vi "AO_mini_stage and shutter control.vi"() -> ()   [LabVIEW 2018]
panel:
  in  "2p shutter":refnum<k7>(container)
  in  "488 shutter":refnum<k7>(container)
  out "Numeric status":dbl
  in  "Flip Mirror":sgl(ring) items=["EMCCD Camera"=-5, "Wavefront sensor"=1]
  in  "stop":bool
  in  "baud rate (9600)":u32=9600
  in  "VISA resource name":refnum<visa-resource-name>="COM5"
  in  "Z step (10=1um)":dbl=2.0
  in  "up":bool
  in  "down":bool
  in  "XY step (10=1um)":u16=50
  in  "back":bool
  in  "front":bool
  in  "left":bool
  in  "right":bool
  # "Sample Stage"
  # "WF switch"
  # "Defocus: +"
  # "Tilt 1/X: +"
  # "Tilt 2/Y: +"
  # "EMCCD: -5"
  # "Wavefront Sensor: 1"
  # "WFS no tilt: X502, Y520 @EMCCD"
  # "Laser Shutter"
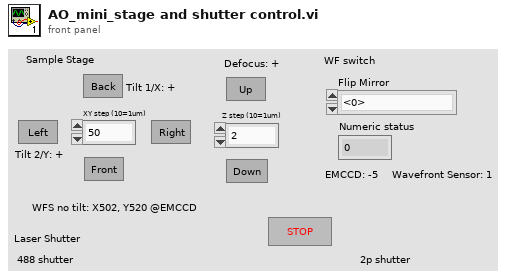
[diagram p1: front panel]
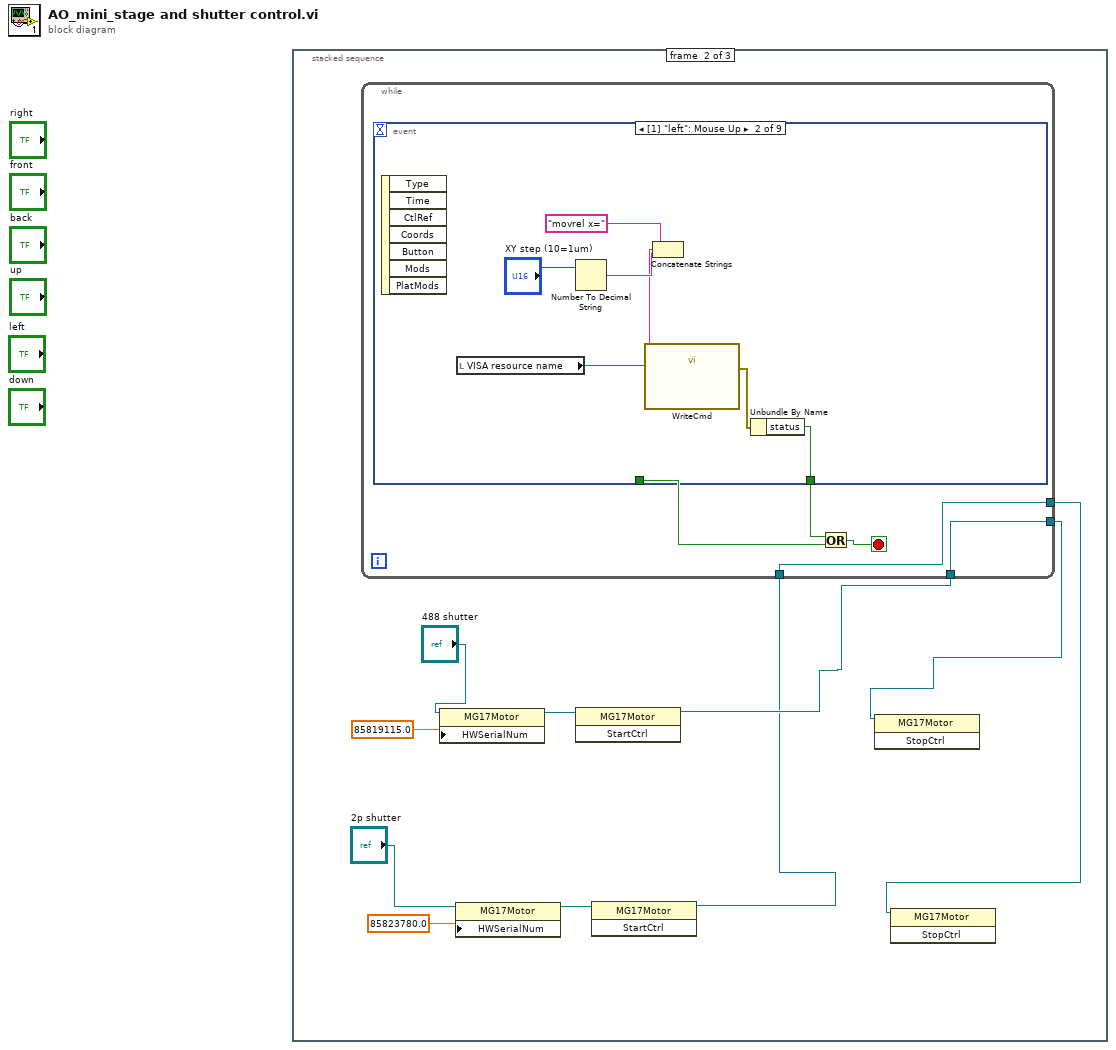
[diagram p0: block diagram]
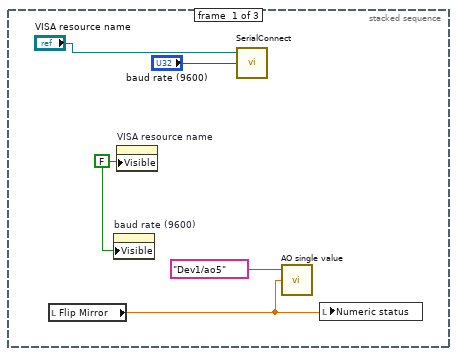
[diagram p2: hidden frame]
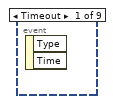
[diagram p3: hidden frame]
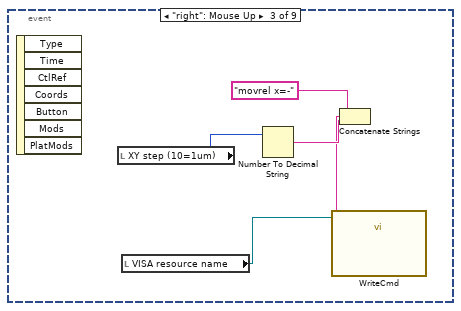
[diagram p4: hidden frame]
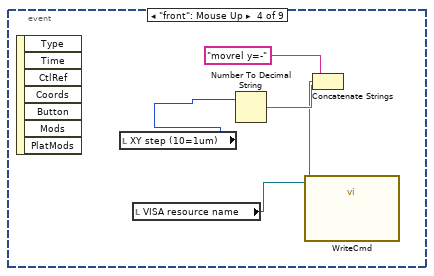
[diagram p5: hidden frame]
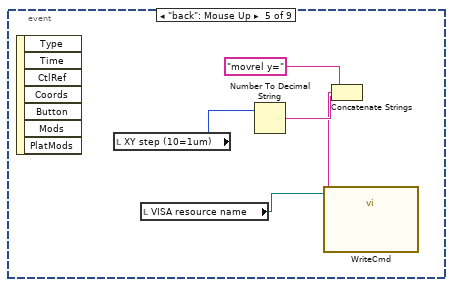
[diagram p6: hidden frame]
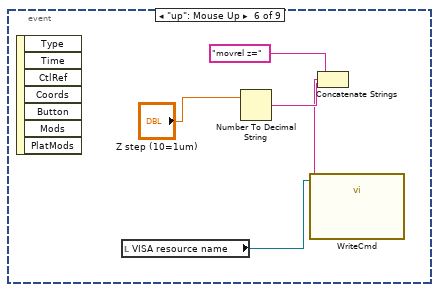
[diagram p7: hidden frame]
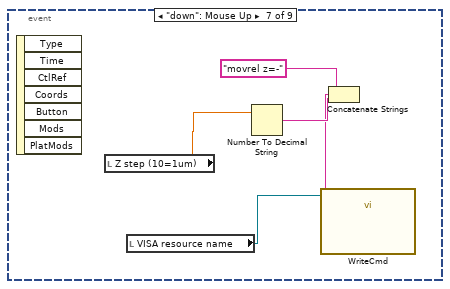
[diagram p8: hidden frame]
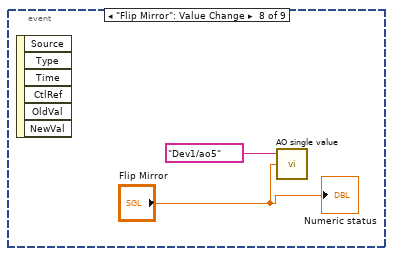
[diagram p9: hidden frame]
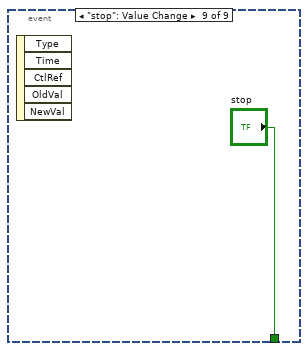
[diagram p10: hidden frame]
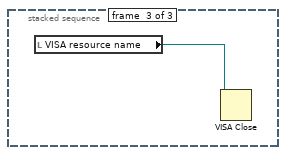
[diagram p11: hidden frame]
diagram:
  n1 = stacked-sequence {
    frame #0 {
      w3 = FALSE ("Visible")
      n2 = local read "Flip Mirror"() -> (w1:sgl)
      n3 = property on="baud rate (9600)" class="DigNum (strict)"("Visible"=w3) -> ()  [unwired: 2 in, 2 out]
      n4 = property on="VISA resource name" class="VISAName"("Visible"=w3) -> ()  [unwired: 2 in, 2 out]
      n5 = call "SerialConnect.vi"("baud rate (9600)"="baud rate (9600)", "VISA resource name"="VISA resource name") -> ()  [unwired: 1 in, 3 out]
      n6 = call "AO single value.vi"("data"=w1, "physical channels"=tag "Dev1/ao5") -> ()  [unwired: 1 in, 1 out]
      n7 = local write "Numeric status"(w1) -> ()
    }
    frame #1 {
      n8 = property class="MG17Motor"(reference="488 shutter", "HWSerialNum"=85819115.0) -> (reference out=w15:refnum<k7>)  [unwired: 1 in, 1 out]
      n9 = property class="MG17Motor"(reference="2p shutter", "HWSerialNum"=85823780.0) -> (reference out=w10:refnum<k7>)  [unwired: 1 in, 1 out]
      n10 = invoke class="MG17Motor" method="StartCtrl"(reference=w15) -> (reference out=w14:refnum<k7>)  [unwired: 2 in, 2 out]
      n11 = invoke class="MG17Motor" method="StartCtrl"(reference=w10) -> (reference out=w7:refnum<k7>)  [unwired: 2 in, 2 out]
      n12 = while {
        tunnel: w14 -> [w17]
        tunnel: [w17] -> w13
        tunnel: w7 -> [w16]
        tunnel: [w16] -> w6
        stop <- w20 stop-if-true
        n13 = event shown="[1] \"left\": Mouse Up" {
          selector: _ -> [_ _ _ _ _ _ _ _ _]
          dyn-events: _ -> [_ _ _ _ _ _ _ _ _]
          timeout: _ -> [_ _ _ _ _ _ _ _ _]
          tunnel: [_ _ _ _ _ _ _ _ "stop"] -> w19
          tunnel: [_ w21 _ _ _ _ _ _ _] -> w18
          event Timeout {
            n14 = event-data() -> ()  [unwired: 1 in, 2 out]
          }
          event "left": Mouse Up {
            n15 = event-data() -> ()  [unwired: 1 in, 7 out]
            n16 = local read "VISA resource name"() -> (w23:refnum<visa-resource-name>)
            n17 = Number To Decimal String(number="XY step (10=1um)") -> (decimal integer string=w25:string)  [unwired: 1 in]
            n18 = Concatenate Strings("movrel x=", w25) -> (w24:string)
            n19 = call "WriteCmd.vi"("Command"=w24, "VISA resource name"=w23) -> ("error"=w22:errorcluster)  [unwired: 1 in]
            n20 = Unbundle By Name(w22) -> ("status"=w21:bool)
          }
          event "right": Mouse Up {
            n21 = event-data() -> ()  [unwired: 1 in, 7 out]
            n22 = local read "XY step (10=1um)"() -> (w28:u16)
            n23 = local read "VISA resource name"() -> (w29:refnum<visa-resource-name>)
            n24 = Number To Decimal String(number=w28) -> (decimal integer string=w31:string)  [unwired: 1 in]
            n25 = Concatenate Strings("movrel x=-", w31) -> (w30:string)
            n26 = call "WriteCmd.vi"("Command"=w30, "VISA resource name"=w29) -> ()  [unwired: 1 in, 1 out]
          }
          event "front": Mouse Up {
            n27 = event-data() -> ()  [unwired: 1 in, 7 out]
            n28 = local read "XY step (10=1um)"() -> (w33:u16)
            n29 = local read "VISA resource name"() -> (w34:refnum<visa-resource-name>)
            n30 = Number To Decimal String(number=w33) -> (decimal integer string=w36:string)  [unwired: 1 in]
            n31 = Concatenate Strings("movrel y=-", w36) -> (w35:string)
            n32 = call "WriteCmd.vi"("Command"=w35, "VISA resource name"=w34) -> ()  [unwired: 1 in, 1 out]
          }
          event "back": Mouse Up {
            n33 = event-data() -> ()  [unwired: 1 in, 7 out]
            n34 = local read "XY step (10=1um)"() -> (w38:u16)
            n35 = local read "VISA resource name"() -> (w39:refnum<visa-resource-name>)
            n36 = Number To Decimal String(number=w38) -> (decimal integer string=w41:string)  [unwired: 1 in]
            n37 = Concatenate Strings("movrel y=", w41) -> (w40:string)
            n38 = call "WriteCmd.vi"("Command"=w40, "VISA resource name"=w39) -> ()  [unwired: 1 in, 1 out]
          }
          event "up": Mouse Up {
            n39 = event-data() -> ()  [unwired: 1 in, 7 out]
            n40 = local read "VISA resource name"() -> (w44:refnum<visa-resource-name>)
            n41 = Number To Decimal String(number="Z step (10=1um)") -> (decimal integer string=w46:string)  [unwired: 1 in]
            n42 = Concatenate Strings("movrel z=", w46) -> (w45:string)
            n43 = call "WriteCmd.vi"("Command"=w45, "VISA resource name"=w44) -> ()  [unwired: 1 in, 1 out]
          }
          event "down": Mouse Up {
            n44 = event-data() -> ()  [unwired: 1 in, 7 out]
            n45 = local read "Z step (10=1um)"() -> (w48:dbl)
            n46 = local read "VISA resource name"() -> (w49:refnum<visa-resource-name>)
            n47 = Number To Decimal String(number=w48) -> (decimal integer string=w51:string)  [unwired: 1 in]
            n48 = Concatenate Strings("movrel z=-", w51) -> (w50:string)
            n49 = call "WriteCmd.vi"("Command"=w50, "VISA resource name"=w49) -> ()  [unwired: 1 in, 1 out]
          }
          event "Flip Mirror": Value Change {
            n50 = event-data() -> ()  [unwired: 1 in, 6 out]
            n51 = call "AO single value.vi"("data"="Flip Mirror", "physical channels"=tag "Dev1/ao5") -> ()  [unwired: 1 in, 1 out]
            "Numeric status" <- "Flip Mirror"
          }
          event "stop": Value Change {
            n52 = event-data() -> ()  [unwired: 1 in, 5 out]
          }
        }
        n53 = Or(x=w18, y=w19) -> (x .or. y?=w20:bool)
      }
      n54 = invoke class="MG17Motor" method="StopCtrl"(reference=w13) -> ()  [unwired: 2 in, 3 out]
      n55 = invoke class="MG17Motor" method="StopCtrl"(reference=w6) -> ()  [unwired: 2 in, 3 out]
    }
    frame #2 {
      n56 = local read "VISA resource name"() -> (w56:refnum<visa-resource-name>)
      n57 = VISA Close(VISA resource name=w56) -> ()  [unwired: 1 in, 1 out]
    }
  }
